vi "TRIG_CHAN_AUX_IPOL.vi"(0 "VISA IN":refnum<visa-resource-name>, 1 "Aux":i32, 2 "Polarity":string(combo)="POS", 5 "error in":errorcluster, 7 "Channel":i32) -> (14 "VISA Out":refnum<visa-resource-name>, 19 "error out":errorcluster)   [LabVIEW 2018, in "PNA-X.lvlib"]
doc: "TRIGger:CHANnel<ch>:AUX<n>:IPOLarity <char> \n(Read-Write) Specifies the polarity of the trigger IN signal to which the PNA will respond. \nParameters \n<ch> Any existing channel number. If unspecified, value is set to 1. \n<n> Rear panel connector used to send or receive signals. \nPNA-X - choose from 1 (AUX TRIG 1) or 2 (AUX TRIG 2) \nAll other models: choose 1. (BNC Trig I/O \nIf unspecified, value is set to 1. \n<char> Choose from: \nPOSitive PNA responds to leading edge or HIGH level \n1890\n\nNEGative PNA responds to trailing edge or LOW level. \nSet Edge or Level triggering using TRIG:CHAN:AUX:TYPE \nExamples TRIG:CHAN:AUX:IPOL POS \ntrigger:channel2:aux2:ipolarity negative \nQuery Syntax TRIGger:CHANnel<ch>:AUX<n>:IPOLarity? \nReturn Type Character \nDefault NEGative"
uses:
  PNA-X.lvlib
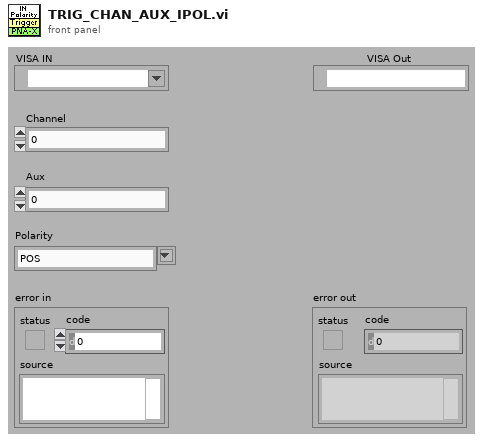
[diagram p1: front panel]
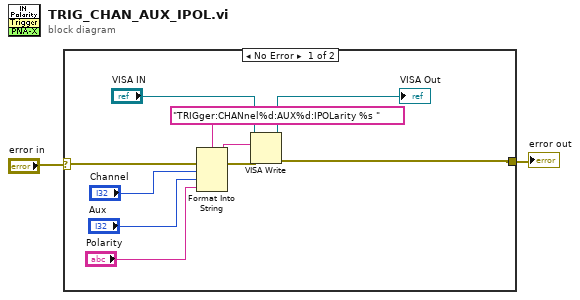
[diagram p0: block diagram]
diagram:
  n1 = case shown="No Error" "error in" {
    selector: "error in" -> [w12 w13]
    tunnel: [w7 w13] -> w1
    frame No Error {
      n2 = Format Into String(format string="TRIGger:CHANnel%d:AUX%d:IPOLarity %s " ("Cmdline"), error in=w12, "Channel", "Aux", "Polarity") -> (resulting string=w10:string, error out=w11:errorcluster)  [unwired: 1 in]
      n3 = VISA Write(VISA resource name="VISA IN", write buffer=w10, error in (no error)=w11) -> (VISA resource name out=→"VISA Out":refnum<visa-resource-name>, error out=w7:errorcluster)  [unwired: 1 out]
    }
    frame Error {
    }
  }
  "error out" <- w1
